vi "CRYMR_Select data.vi"(1 "Tolerance":u16(ring) items=["Single Point", "Absolute Limits", "Floating Limits", "Floating Data", "Aligned Limits", "Aligned Data", "Voltmeter", "Frequency Shift"], 2 "Data":cluster{"Hz":dbl, "dB":dbl}[](array[cluster])=[{"Hz"=2.3010299956639813, "dB"=2.9}, {"Hz"=2.6989700043360187, "dB"=3.5}, {"Hz"=3.0, "dB"=5.0}, {"Hz"=3.3010299956639813, "dB"=6.0}, {"Hz"=3.6989700043360187, "dB"=4.0}] {"dB" format="%.2f"; "Hz" format="%.2f"}, 3 "Lower Limit":cluster{"Hz":dbl, "y":dbl}[](array[cluster])=[{"Hz"=2.6020599913279625, "y"=0.5}, {"Hz"=3.0, "y"=3.5}, {"Hz"=3.4771212547196626, "y"=1.5}] {"Hz" format="%.2f"; "y" format="%.2f"}, 4 "Upper Limit":cluster{"Hz":dbl, "y":dbl}[](array[cluster])=[{"Hz"=2.4771212547196626, "y"=4.0}, {"Hz"=3.0, "y"=6.5}, {"Hz"=3.6020599913279625, "y"=5.0}, {"Hz"=4.8, "y"=4.5}, {"Hz"=4.0, "y"=0.0}] {"Hz" format="%.2f"; "y" format="%.2f"}) -> (0 "Data Out":cluster{dbl, dbl}[](array[cluster])=[{2.4771212547196626, 3.1655042296098563}, {2.6020599913279625, 3.353882478419618}, {3.0, 5.0}, {3.4771212547196626, 5.1149859013004795}, {3.6020599913279625, 4.487058405267939}] {"?" format="%.2f"; "?" format="%.2f"})   [LabVIEW 2013]
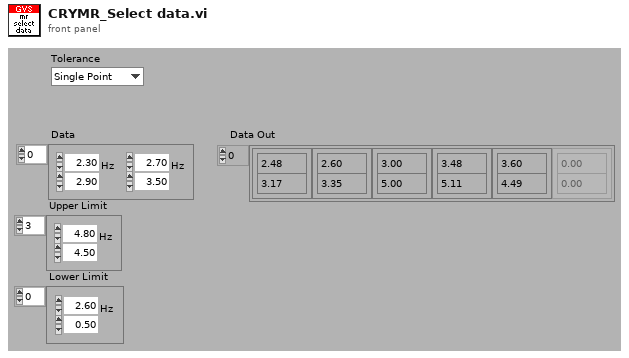
[diagram p1: front panel]
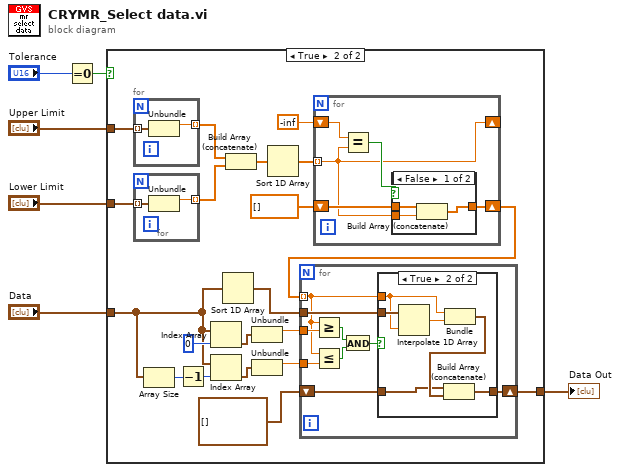
[diagram p0: block diagram]
diagram:
  n1 = Equal To 0?(x="Tolerance") -> (x = 0?=w5:bool)
  n2 = case shown="True" w5 {
    tunnel: "Upper Limit" -> [_ w23]
    tunnel: "Lower Limit" -> [_ w22]
    tunnel: "Data" -> [w7 w9]
    tunnel: [w7 w10] -> w1
    frame False {
    }
    frame True {
      n3 = for {
        tunnel: [w56] -> w27 mode=indexing
        tunnel: w23 -> [w55] mode=indexing
        n4 = Unbundle(w55) -> ("Hz"=w56:dbl)  [unwired: 1 out]
      }
      n5 = for {
        tunnel: [w54] -> w26 mode=indexing
        tunnel: w22 -> [w53] mode=indexing
        n6 = Unbundle(w53) -> ("Hz"=w54:dbl)  [unwired: 1 out]
      }
      n7 = Array Size(array=w9) -> (size(s)=w18:i32)
      n8 = Decrement(x=w18) -> (x-1=w14:i32)
      n9 = Index Array(array=w9, index=0) -> (element=w15:cluster{"Hz":dbl, "dB":dbl})
      n10 = Index Array(array=w9, index=w14) -> (element=w16:cluster{"Hz":dbl, "dB":dbl})
      n11 = Sort 1D Array(array=w9) -> (sorted array=w8:cluster{"Hz":dbl, "dB":dbl}[])
      n12 = Build Array (concatenate)(w27, w26) -> (w21:dbl[])
      n13 = Unbundle(w15) -> ("Hz"=w13:dbl)  [unwired: 1 out]
      n14 = Unbundle(w16) -> ("Hz"=w12:dbl)  [unwired: 1 out]
      n15 = Sort 1D Array(array=w21) -> (sorted array=w24:dbl[])
      n16 = for {
        shift-right: [w44] -> _
        shift-left: -inf -> [w48]
        tunnel: w24 -> [w44] mode=indexing
        shift-right: [w46] -> w19
        shift-left: dbl[] [] -> [w45]
        n17 = Equal?(x=w48, y=w44) -> (x = y?=w47:bool)
        n18 = case shown="False" w47 {
          tunnel: w45 -> [w50 w52]
          tunnel: [w51 w52] -> w46
          tunnel: w44 -> [w49 _]
          frame False {
            n19 = Build Array (concatenate)(w50, w49) -> (w51:dbl[])
          }
          frame True {
          }
        }
      }
      n20 = for {
        tunnel: w19 -> [w30] mode=indexing
        tunnel: w8 -> [w31]
        tunnel: w13 -> [w36]
        tunnel: w12 -> [w35]
        shift-right: [w28] -> w10
        shift-left: cluster{dbl, dbl}[] [] -> [w29]
        n21 = Greater Or Equal?(x=w30, y=w36) -> (x >= y?=w34:bool)
        n22 = Less Or Equal?(x=w30, y=w35) -> (x <= y?=w33:bool)
        n23 = And(x=w34, y=w33) -> (x .and. y?=w32:bool)
        n24 = case shown="True" w32 {
          tunnel: w31 -> [_ w42]
          tunnel: w30 -> [_ w41]
          tunnel: w29 -> [w37 w38]
          tunnel: [w37 w40] -> w28
          frame False {
          }
          frame True {
            n25 = Interpolate 1D Array(1:w41, 2:w42) -> (0:w43:dbl)
            n26 = Bundle(w41, w43) -> (w39:cluster{dbl, dbl})  [unwired: 1 in]
            n27 = Build Array (concatenate)(w38, w39) -> (w40:cluster{dbl, dbl}[])
          }
        }
      }
    }
  }
  "Data Out" <- w1
